vi "Example Simple.vi"() -> ()   [LabVIEW 2013]
uses:
  C:/tf/play/labview/Tinkerforge.dll
  Tinkerforge.dll
panel:
  out "timestamp (ms)":i64
  out "weekday":u8
  out "centisecond":u8
  out "second":u8
  out "minute":u8
  out "hour":u8
  out "day":u8
  out "month":u8
  out "year":i32
  in  "uid":string="XYZ"
  in  "port":i32=4223
  in  "host":string="localhost"
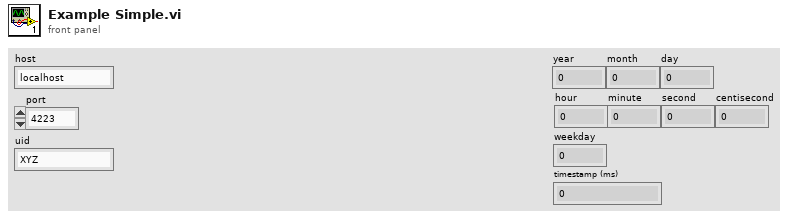
[diagram p1: front panel]
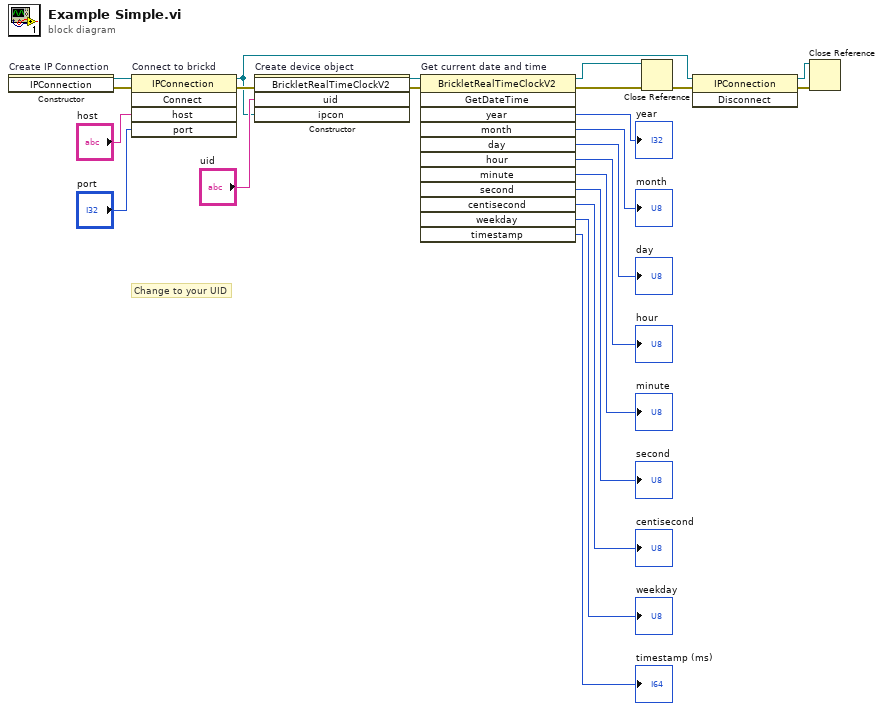
[diagram p0: block diagram]
diagram:
  # "Change to your UID"
  n1 = constructor on="Create IP Connection" class="IPConnection"() -> (reference out=w23:refnum<k24>, error out=w12:errorcluster)  [unwired: 3 in, 1 out]
  n2 = invoke on="Connect to brickd" class="IPConnection" method="Connect"(reference=w23, error in=w12, "host"="host", "port"="port") -> (reference out=w14:refnum<k24>, error out=w19:errorcluster)  [unwired: 1 in, 3 out]
  n3 = constructor on="Create device object" class="BrickletRealTimeClockV2"(error in=w19, "uid"="uid", "ipcon"=w14) -> (reference out=w17:refnum<k24>, error out=w18:errorcluster)  [unwired: 2 in, 3 out]
  n4 = invoke on="Get current date and time" class="BrickletRealTimeClockV2" method="GetDateTime"(reference=w17, error in=w18) -> (reference out=w3:refnum<k24>, error out=w2:errorcluster, "year"=→"year":i32, "month"=→"month":u8, "day"=→"day":u8, "hour"=→"hour":u8, "minute"=→"minute":u8, "second"=→"second":u8, "centisecond"=→"centisecond":u8, "weekday"=→"weekday":u8, "timestamp"=→"timestamp (ms)":i64)  [unwired: 10 in, 1 out]
  n5 = Close Reference(reference=w3, error in (no error)=w2) -> (error out=w16:errorcluster)
  n6 = invoke class="IPConnection" method="Disconnect"(reference=w14, error in=w16) -> (reference out=w13:refnum<k24>, error out=w15:errorcluster)  [unwired: 1 in, 1 out]
  n7 = Close Reference(reference=w13, error in (no error)=w15) -> ()  [unwired: 1 out]
